vi "HIL Simulation and Testing - State Machine.vi"() -> ()   [LabVIEW 2021]
uses:
  <vilib>/Simulation/Scripting/Companion Diagram/SimConfigNode/SimParams.ctl
  <vilib>/Simulation/Scripting/Companion Diagram/SimConfigNode/_simSolvers.ctl
  <vilib>/Simulation/Implementation/Shared/SIMSCR Execution Mode.ctl
  <vilib>/Simulation/Param Hierarchy/Typedefs/SIMPH Param Control Actions.ctl
  <vilib>/Simulation/Implementation/Shared/NILVSim_ParamChanged.vi
  <vilib>/Simulation/Implementation/Shared/NILVSIM_BeginStep.vi
  <vilib>/Simulation/Implementation/Shared/NILVSim_Manager.vi
  <vilib>/Utility/error.llb/Clear Errors.vi
  <vilib>/Simulation/Implementation/Shared/NILVSim_FinalizeModel.vi
  <vilib>/Simulation/Implementation/Shared/SIM Unbundle Sim Info.vi
  <vilib>/Simulation/Implementation/Shared/NILVSim_Initialize.vi
  <vilib>/Simulation/Utility/Implementation/NILVSim Get Time and IsAcceptedStep.vi
  <vilib>/Simulation/Implementation/Shared/SIMSH Read Queue.vi
  <vilib>/Simulation/Implementation/Shared/NILVSim_GetModelError.vi
  <vilib>/Simulation/Implementation/Shared/SIM Bundle Sim Info.vi
  <vilib>/Simulation/Implementation/XNodeFramework/SimXNode/SimX.xnode
  Blackbox/Air Heater Black Box Model.vi
  <vilib>/Simulation/Scripting/Companion Diagram/SimConfigNode/SimDog.xnode
  <vilib>/Simulation/Implementation/Shared/NI_SIM_Implementation.lvlib
panel:
  out "Control Value [V]":dbl format="%.2g"
  out "Temperature [°C]":dbl format="%.1g"
  out "Control Chart":dbl(graph)=1.1724378087907898
  out "Measurement Chart":dbl(graph)
  in  "Stop":bool
  # "Note! The Setpoint/Set Value (SV) is set on the Fuji PXG5 Hardware"
  # "Process Value (PV)"
  # "Manipulated Value (MV)"
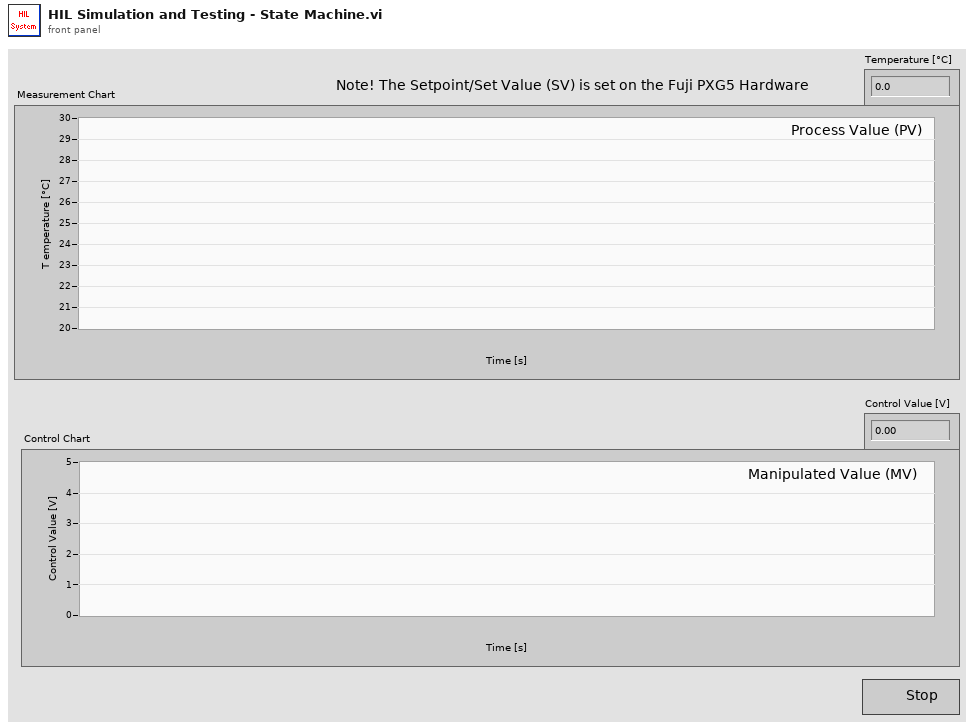
[diagram p1: front panel]
types:
  T1 = enum16{"Simulate to Completion", "Single Time-Step Simulation (Fixed Step Only)"}
  T2 = typedef "SIMSCR Execution Mode.ctl" = enum16{"Simulate to Completion", "Single Time-Step Simulation (Fixed Step Only)"}
  T3 = typedef "SIMPH Param Control Actions.ctl" = enum16{"get params", "set params"}
  T4 = cluster{"SIMSH Sim Time":dbl, "Linear Scaling with Points.vi 2":cluster{"Output":dbl}, "Select":cluster{"s? t:f":dbl}, "Summation 3":cluster{"Result":dbl}, "Square Root":cluster{"sqrt(x)":dbl}, "Gaussian White Noise PtByPt.vi":cluster{"Gaussian white noise":dbl}, "Integrator":cluster{"output":dbl}, "Multiplication":cluster{"Result":dbl}, "Summation":cluster{"Result":dbl}, "Multiplication 2":cluster{"Result":dbl}, "Transport Delay":cluster{"output":dbl}, "Summation 2":cluster{"Result":dbl}}
  T5 = typedef "SimParams.ctl" = cluster{"Initial Time (s)":dbl, "Final Time (s)":dbl, "Step Size (s)":dbl, "ODE Solver":T6, "Minimum Step Size (s)":dbl, "Maximum Step Size (s)":dbl, "Relative Tolerance":dbl, "Absolute Tolerance":dbl, "Software Timing":bool, "Initial Step Size (s)":dbl, "Automatic Fixed Step Size?":bool, "Automatic Discrete Step Size?":bool, "Discrete Step Size (s)":dbl, "Calculate using Time Step":bool, "Solver Wired?":bool, "Prev.Frm.Expected End":u64, "Prev.Frm.Actual End":u64, "Prev.Frm.Finished Late?":bool, "Prev.Iter.Expected End":u64, "Prev.Iter.Actual End":u64, "Prev.Iter.Finished Late?":bool, "Expected Iteration Start":u64, "Actual Iteration Start":u64, "Expected Frame Start":u64, "Actual Frame Start":u64, "Source Name":string, "Name":string, "Period":i64, "Deadline":i64, "Offset":i64, "Start":i64, "Priority":i32, "Timeout":i32, "Processor":i32, "Mode":enum32{"No Change", "Process missed periods, maintain original phase", "Discard missed periods, maintain original phase", "Process missed periods, ignore original phase", "Discard missed periods, ignore original phase"}, "Wakeup reason":enum32{"Normal", "Aborted", "Asynchronous wakeup", "Timing source error", "Timed loop error", "Timeout"}, "Error":errorcluster, "Source Type":string, "Secondary Source Type":string, "Global End Time":u64, "Global Start Time":u64, "Full Solver Reset":bool, "Execution Mode":T2, "Nan/Inf Check":bool, "Custom Solver Library":string, "Solver Is Variable":bool, "custom solver name":string, "Signal Collection Decimation":u32}
  T6 = typedef "_simSolvers.ctl" = enum16{"Runge-Kutta 1 (Euler)", "Runge-Kutta 2", "Runge-Kutta 3", "Runge-Kutta 4", "Runge-Kutta 23 (variable)", "Runge-Kutta 45 (variable)", "BDF (variable)", "Adams-Moulton (variable)", "Rosenbrock (variable)", "Discrete States Only", "SDIRK 4 (variable)", "Radau 5 (variable)", "Radau 9 (variable)", "Radau 13 (variable)", "Radau [Variable Order] (variable)", "Gear's Method (variable)", "Linearizer", "State Query", "Trim Eval", "Custom Solver"}
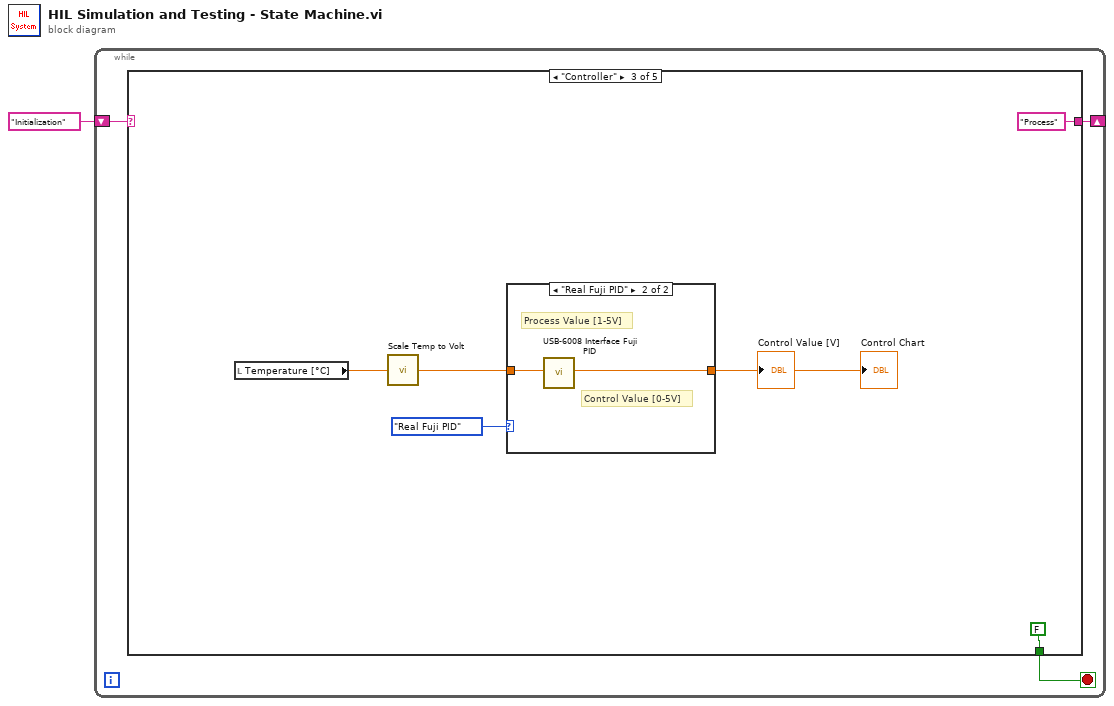
[diagram p0: block diagram]
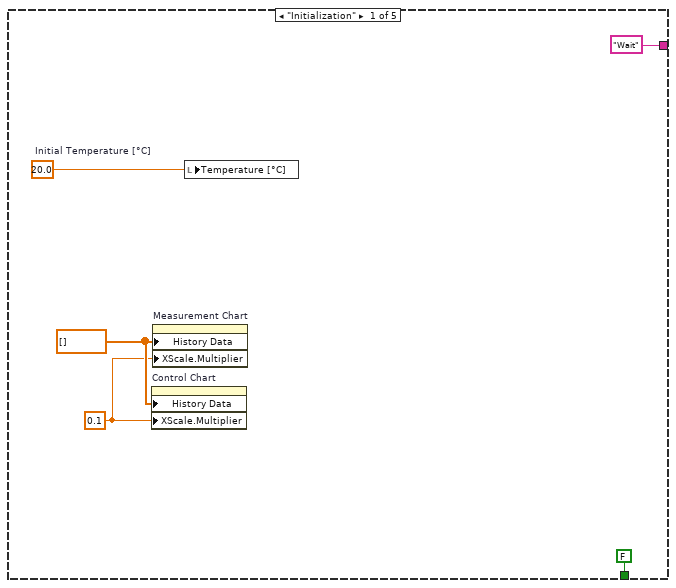
[diagram p2: hidden frame]
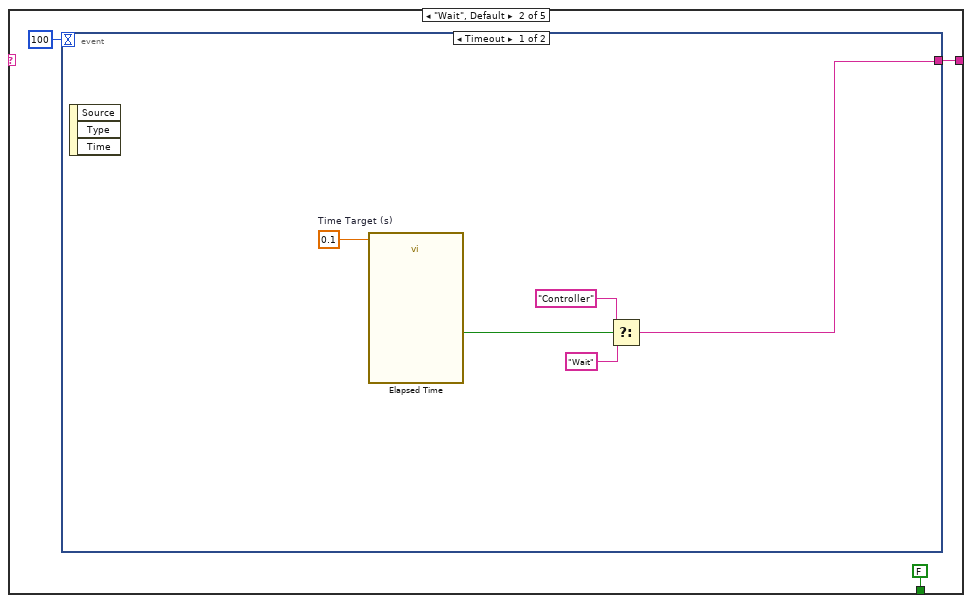
[diagram p3: hidden frame]
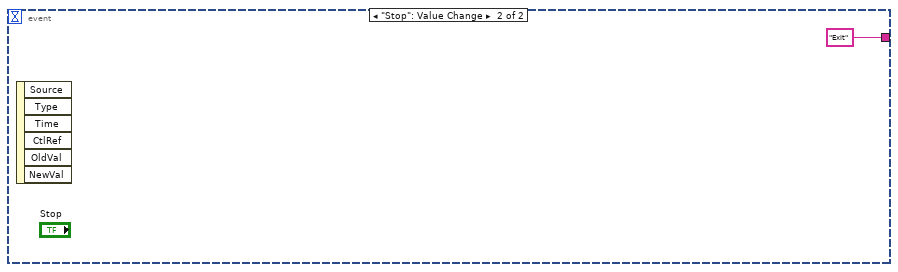
[diagram p4: hidden frame]
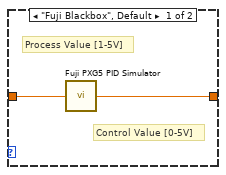
[diagram p5: hidden frame]
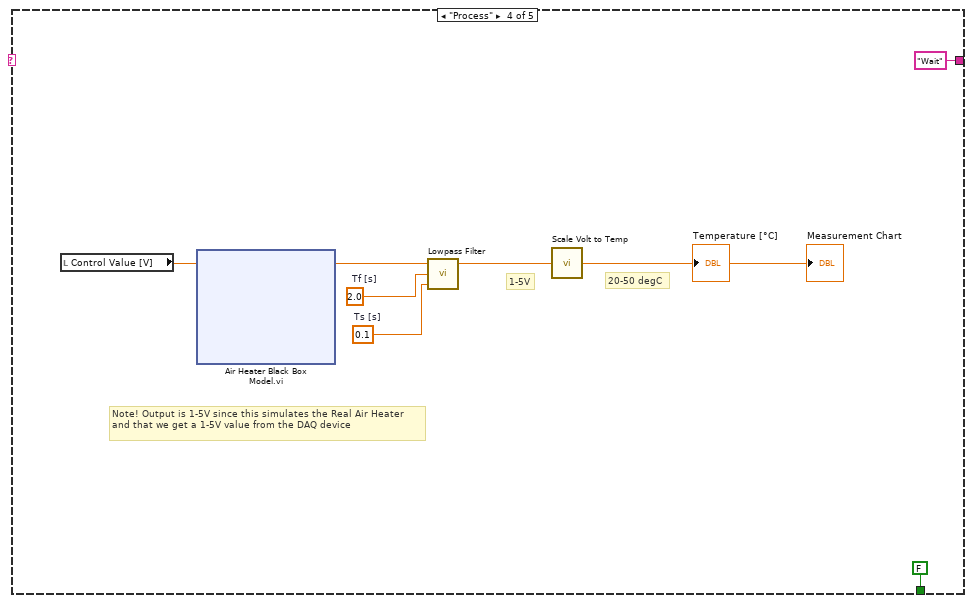
[diagram p6: hidden frame]
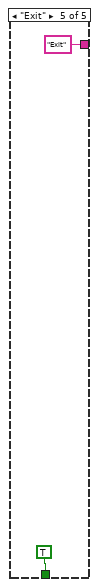
[diagram p7: hidden frame]
diagram:
  n1 = while {
    shift-right: [w3] -> _
    shift-left: "Initialization" -> [w4]
    stop <- w2 stop-if-true
    n2 = case shown="\"Controller\"" w4 {
      tunnel: ["Wait" w10 "Process" "Wait" "Exit"] -> w3
      tunnel: [FALSE FALSE FALSE FALSE TRUE] -> w2
      frame "Initialization" {
        w5 = 20.0  # Initial Temperature [°C]
        w6 = 0.1 ("X Scale.Offset and Multiplier:Multiplier")
        w7 = dbl[] [] ("History Data")
        n3 = property on="Control Chart" class="WFChart (strict)"("History Data"=w7, "XScale.Multiplier"=w6) -> ()  [unwired: 2 in, 2 out]
        n4 = property on="Measurement Chart" class="WFChart (strict)"("History Data"=w7, "XScale.Multiplier"=w6) -> ()  [unwired: 2 in, 2 out]
        n5 = local write "Temperature [°C]"(w5) -> ()
      }
      frame "Wait", Default {
        n6 = event shown="[0] Timeout" {
          selector: _ -> [_ _]
          dyn-events: _ -> [_ _]
          timeout: 100 -> [_ _]
          tunnel: [w13 "Exit"] -> w10
          event Timeout {
            w14 = 0.1  # Time Target (s)
            n7 = event-data() -> ()  [unwired: 1 in, 3 out]
            n8 = call "Elapsed Time"("Time Target (s)"=w14) -> ("Time has Elapsed"=w17:bool)  [unwired: 11 in, 7 out]
            n9 = Select(t="Controller", s=w17, f="Wait") -> (s? t:f=w13:string)
          }
          event "Stop": Value Change {
            n10 = event-data() -> ()  [unwired: 1 in, 6 out]
          }
        }
      }
      frame "Controller" {
        n11 = local read "Temperature [°C]"() -> (w19:dbl)
        n12 = call "Scale Temp to Volt.vi"("Input Value [20-50degC]"=w19) -> ("Output Value [1-5V]"=w22:dbl)
        n13 = case shown="\"Real Fuji PID\"" enum16{"Fuji Blackbox", "Real Fuji PID"}."Real Fuji PID" ("Enum") {
          tunnel: [w26 w27] -> w21
          tunnel: w22 -> [w25 w28]
          frame "Fuji Blackbox", Default {
            # "Process Value [1-5V]"
            # "Control Value [0-5V]"
            n14 = call "Fuji PXG5 PID Simulator.vi"("Input (1-5V)"=w25) -> ("Output (0-5V)"=w26:dbl)
          }
          frame "Real Fuji PID" {
            # "Process Value [1-5V]"
            # "Control Value [0-5V]"
            n15 = call "USB-6008 Interface Fuji PID.vi"("Process Value  [1-5V]"=w28) -> ("Control Value [0-5V]"=w27:dbl)
          }
        }
        "Control Chart" <- w21
        "Control Value [V]" <- w21
      }
      frame "Process" {
        w31 = 0.1  # Ts [s]
        w30 = 2.0  # Tf [s]
        # "Note! Output is 1-5V since this simulates the Real Air Heater and that we get a 1-5V value from the DAQ device"
        # "1-5V"
        # "20-50 degC"
        n16 = local read "Control Value [V]"() -> (w29:dbl)
        n17 = xnode "Air Heater Black Box Model.vi"("Control Signal [0-5V]"=w29) -> ("Tout [1-5V]"=w32:dbl)  [unwired: 2 in, 1 out]
        n18 = call "Lowpass Filter.vi"("Ts [s]"=w31, "Tf [s]"=w30, "Filter Input"=w32) -> ("Filter Output"=w33:dbl)
        n19 = call "Scale Volt to Temp.vi"("Input Value [1-5V]"=w33) -> ("Output Value [20-50degC]"=→"Measurement Chart" →"Temperature [°C]":dbl)
      }
      frame "Exit" {
      }
    }
  }
